vi "Table Value To 1D I64.vi"(11 "Table Ref In":refnum<vi>) -> (1 "I64 Out":i64[](array[numeric]), 3 "Table Ref Out":refnum<vi>)   [LabVIEW 2024]
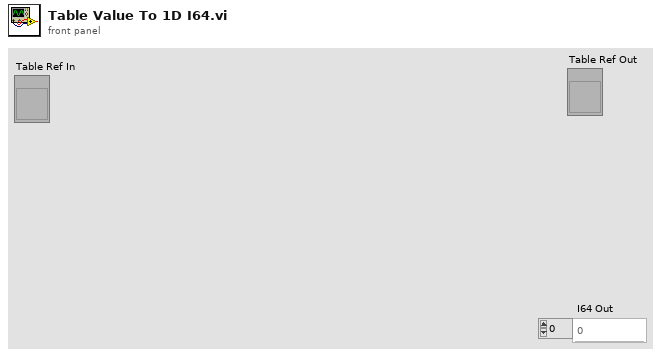
[diagram p1: front panel]
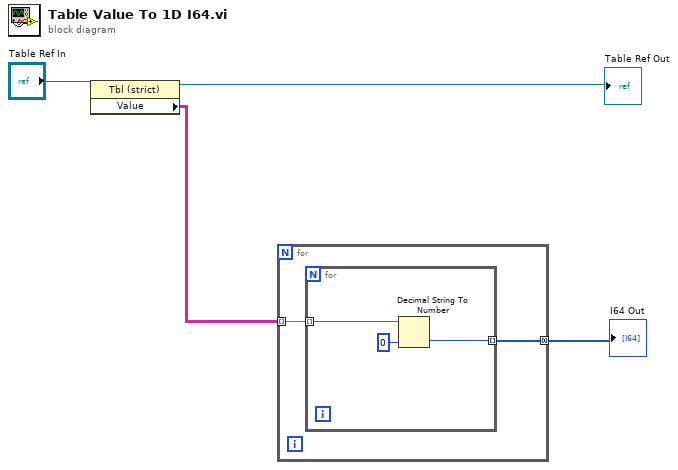
[diagram p0: block diagram]
diagram:
  n1 = property class="Tbl (strict)"(reference="Table Ref In") -> (reference out=→"Table Ref Out":refnum<vi>, "Value"=w2:string[][])  [unwired: 1 in, 1 out]
  n2 = for {
    tunnel: w2 -> [w6] mode=indexing
    tunnel: [w5] -> w1 mode=concatenating
    n3 = for {
      tunnel: w6 -> [w9] mode=indexing
      tunnel: [w7] -> w5 mode=indexing
      n4 = Decimal String To Number(string=w9, default (0L)=i64 0 ("default (0 I32)")) -> (number=w7:i64)  [unwired: 1 in, 1 out]
    }
  }
  "I64 Out" <- w1
